vi "Update UI Data.vi"(0 "Stage in":refnum<class "Stage.lvclass">, 5 "Stage X Position":dbl format="%#_13g", 7 "Stage Y Position":dbl format="%#_13g", 9 "Stage Z Position":dbl format="%#_13g", 11 "error in (no error)":errorcluster) -> (4 "Stage out":refnum<class "Stage.lvclass">, 15 "error out":errorcluster)   [LabVIEW 2020, in "Stage.lvlib" / "Stage.lvclass"]
uses:
  Stage.lvclass
  Stage.lvclass/Stage.ctl
  Stage Controller Messages/Update UI Msg/Update UI Msg.lvclass/Update UI Msg.ctl
  <vilib>/ActorFramework/Message Enqueuer/Message Enqueuer.lvclass/Message Enqueuer.ctl
  <vilib>/ActorFramework/Message Enqueuer/Enqueue.vi
  Stage Controller Messages/Update UI Msg/Update UI Msg.lvclass
  C:/Program Files/National Instruments/LabVIEW 2020/vi.lib/ActorFramework/Message/Message.lvclass
  <vilib>/ActorFramework/Message Priority Queue/Priority Enqueue.vi
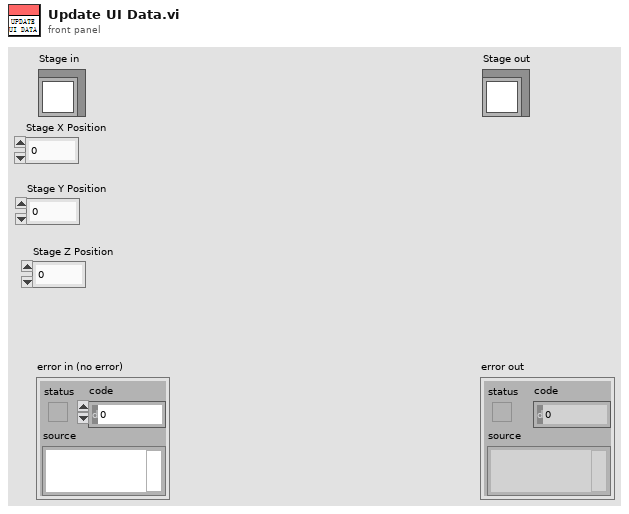
[diagram p1: front panel]
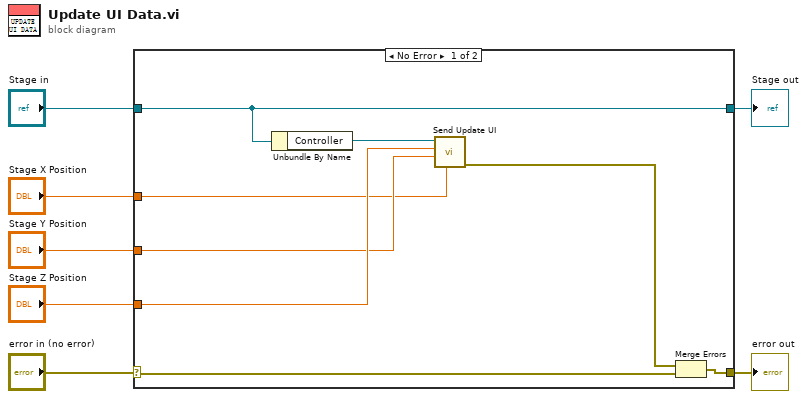
[diagram p0: block diagram]
diagram:
  n1 = case shown="No Error" "error in (no error)" {
    selector: "error in (no error)" -> [w10 w17]
    tunnel: [w9 w17] -> w6
    tunnel: [w15 w16] -> w4
    tunnel: "Stage in" -> [w15 w16]
    tunnel: "Stage Z Position" -> [w13 _]
    tunnel: "Stage Y Position" -> [w12 _]
    tunnel: "Stage X Position" -> [w11 _]
    frame No Error {
      n2 = Unbundle By Name(w15) -> ("Controller"=w14:refnum<class "Message Enqueuer.lvclass">)
      n3 = call "Send Update UI.vi"("Stage X Position"=w11, "Stage Y Position"=w12, "Stage Z Position"=w13, "Message Enqueuer"=w14) -> ("error out"=w8:errorcluster)  [unwired: 6 in, 1 out]
      n4 = Merge Errors(w8, w10) -> (w9:errorcluster)
    }
    frame Error {
    }
  }
  "error out" <- w6
  "Stage out" <- w4
